vi "escribeListaDePruebas.vi"(8 "error in (no error)":errorcluster, 11 "Sonometro in":refnum<class "Sonometro.lvclass">) -> (0 "error out":errorcluster, 3 "Sonometro out":refnum<class "Sonometro.lvclass">)   [LabVIEW 2019, in "Sonometro.lvclass"]
uses:
  Sonometro.lvclass
  D:/REPO/GitHub/procal/Equipo/Equipo/Equipo.lvclass
  Sonometro.lvclass/Sonometro.ctl
  Base de Datos/Base de Datos.lvclass
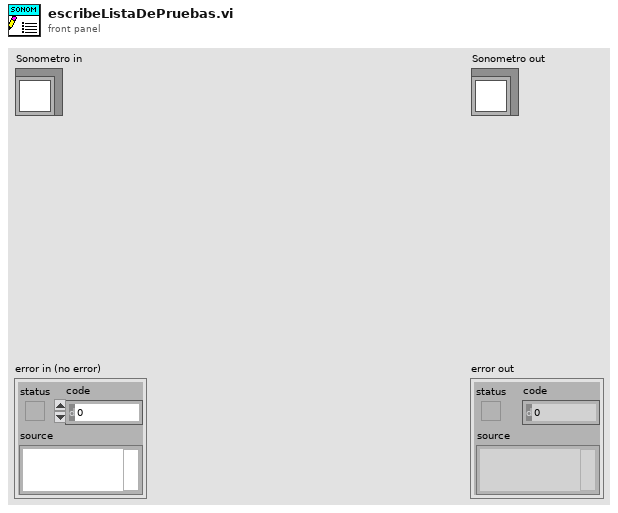
[diagram p1: front panel]
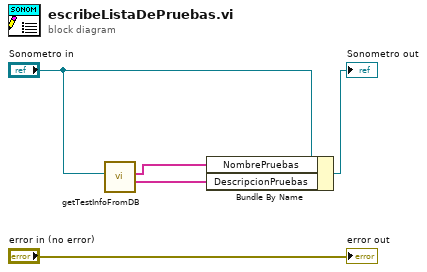
[diagram p0: block diagram]
diagram:
  n1 = call "getTestInfoFromDB.vi"("Equipo.lvclass"="Sonometro in") -> ("DescripcionPruebas"=w5:string[], "NombrePruebas"=w1:string[])  [unwired: 7 in, 2 out]
  n2 = Bundle By Name(cluster="Sonometro in", "NombrePruebas"=w1, "DescripcionPruebas"=w5) -> (→"Sonometro out":refnum<class "Sonometro.lvclass">)
  "error out" <- "error in (no error)"
